vi "Pedestal.vi"(2 "Varray":dbl[](array[numeric]), 3 "ArraySize":i32) -> (0 "Average":dbl, 1 "L-R":dbl)   [LabVIEW 2018]
uses:
  <vilib>/Analysis/NI_AALBase.lvlib
panel:
  # "Calculates pedestal average and difference"
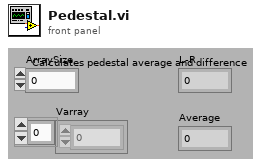
[diagram p1: front panel]
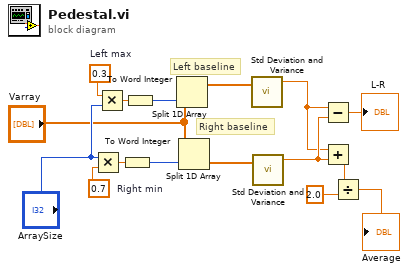
[diagram p0: block diagram]
diagram:
  w3 = 0.3  # Left max
  w1 = 0.7  # Right min
  # "Right baseline"
  # "Left baseline"
  n1 = Multiply(x="ArraySize", y=w1) -> (x*y=w2:dbl)
  n2 = Multiply(x=w3, y="ArraySize") -> (x*y=w4:dbl)
  n3 = To Word Integer(number=w2) -> (16bit integer=w8:i16)
  n4 = To Word Integer(number=w4) -> (16bit integer=w5:i16)
  n5 = Split 1D Array(array="Varray", index=w5) -> (first subarray=w6:dbl[])  [unwired: 1 out]
  n6 = Split 1D Array(array="Varray", index=w8) -> (second subarray=w9:dbl[])  [unwired: 1 out]
  n7 = call <vilib>:"Std Deviation and Variance.vi"("X"=w6) -> ("mean"=w13:dbl)  [unwired: 1 in, 2 out]
  n8 = call <vilib>:"Std Deviation and Variance.vi"("X"=w9) -> ("mean"=w14:dbl)  [unwired: 1 in, 2 out]
  n9 = Subtract(x=w13, y=w14) -> (x-y=→"L-R":dbl)
  n10 = Add(x=w13, y=w14) -> (x+y=w15:dbl)
  n11 = Divide(x=w15, y=2.0) -> (x/y=→"Average":dbl)
